vi "EnableEqualization.vi"(8 "error in (no error)":errorcluster, 10 "Enable/Disable":bool, 11 "reference in":refnum<class "sim_MmW.lvclass">) -> (0 "error out":errorcluster, 3 "reference out":refnum<class "sim_MmW.lvclass">)   [LabVIEW 2019, in "sim_MmW.lvclass"]
doc: "Enables or disabled signal calibration"
uses:
  sim_MmW.lvclass
  C:/Barkhausen mmWave radar/Development/LV/Barkhausen mmWave hardware control/Host/SubVIs/mmWave instrument_class/mmWave instrument.lvclass
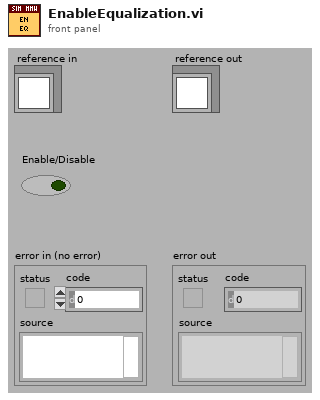
[diagram p1: front panel]
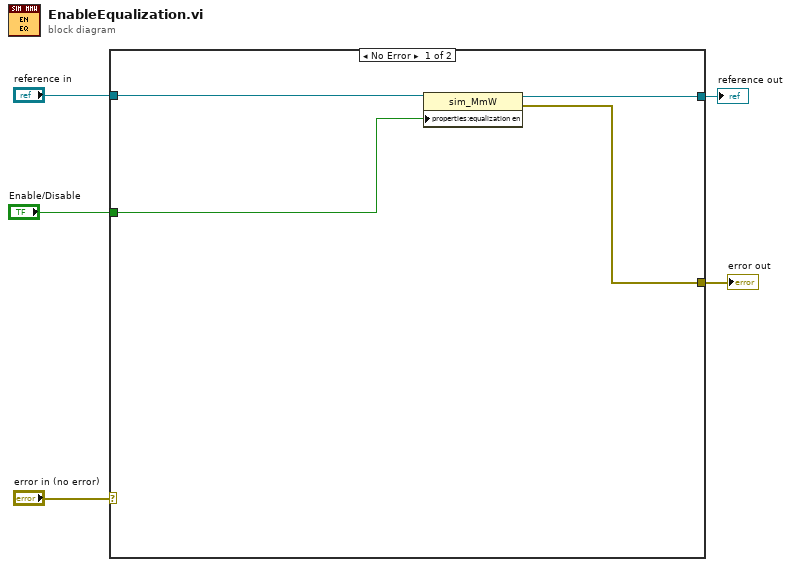
[diagram p0: block diagram]
diagram:
  n1 = case shown="No Error" "error in (no error)" {
    selector: "error in (no error)" -> [_ w11]
    tunnel: [w6 w11] -> w4
    tunnel: [w7 w10] -> w2
    tunnel: "reference in" -> [w8 w10]
    tunnel: "Enable/Disable" -> [w9 _]
    frame No Error {
      n2 = property class="sim_MmW"(reference=w8, "properties:equalization en"=w9) -> (reference out=w7:refnum<class "sim_MmW.lvclass">, error out=w6:errorcluster)  [unwired: 1 in]
    }
    frame Error {
    }
  }
  "error out" <- w4
  "reference out" <- w2
